vi "DSE6_x_defaut.vi"(2 "tmax":dbl, 3 "Loi Expo.":T1) -> (1 "X (Défaut)":T2)   [LabVIEW 2010, in "lv_02.lvlib"]
uses:
  lv_01/do_serie-c.ctl
  p_5E6_Lexp.ctl
  lv_01/0002-03.vi
  lv_02.lvlib
  lv_01/lv_01.lvlib
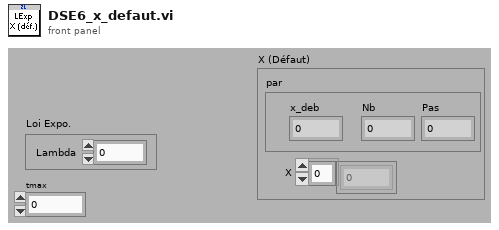
[diagram p1: front panel]
types:
  T1 = typedef "lv_02.lvlib/p_5E6_Lexp.ctl" = cluster{"Lambda":dbl}
  T2 = typedef "lv_01.lvlib/do_serie-c.ctl" = cluster{"X":dbl[], "par":cluster{"x_deb":dbl, "Pas":dbl, "Nb":dbl}}
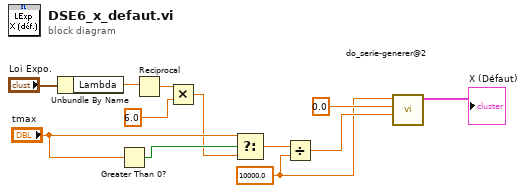
[diagram p0: block diagram]
diagram:
  w1 = 10000.0 ("y")
  n1 = Unbundle By Name("Loi Expo.") -> ("Lambda"=w7:dbl)
  n2 = Greater Than 0?(x="tmax") -> (x > 0?=w10:bool)
  n3 = Reciprocal(x=w7) -> (1/x=w6:dbl)
  n4 = Multiply(x=w6, y=6.0) -> (x*y=w4:dbl)
  n5 = Select(t="tmax", s=w10, f=w4) -> (s? t:f=w8:dbl)
  n6 = Divide(x=w8, y=w1) -> (x/y=w2:dbl)
  n7 = call-poly "do_serie-generer@2.vi"("Pas"=w2, "x_deb"=0.0, "Nb"=w1) -> ("sér. (s)"=→"X (Défaut)":T2)  [unwired: 8 in]
